vi "SmoothImage.vi"(0 "sector array in":cdb[][](array[numeric]) format="%.2f", 1 "Override min fill?":bool, 2 "Av size":i32=3, 3 "Min value":dbl format="%.2f") -> (4 "Smoothed Median":dbl[][](array[numeric]) format="%.2f", 5 "Smoothed Sector w/Ave":cdb[][](array[numeric]) format="%.2f", 6 "Var Array":dbl[][](array[numeric]), 7 "Soothed Sector w/ Max neighbor":dbl[][](array[numeric]) format="%.2f")   [LabVIEW 2022 SP3]
uses:
  <vilib>/Analysis/NI_AALBase.lvlib
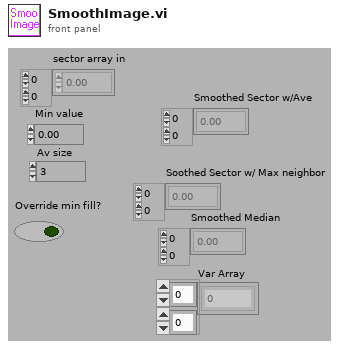
[diagram p1: front panel]
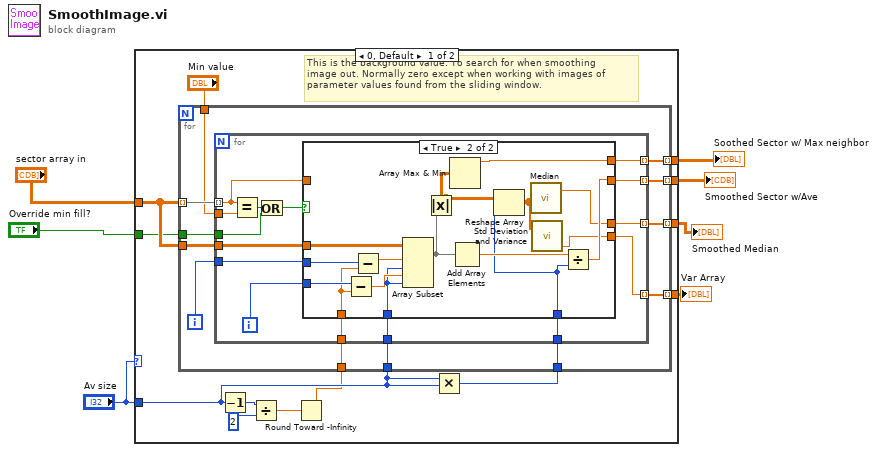
[diagram p0: block diagram]
diagram:
  n1 = case shown="0, Default" "Av size" {
    tunnel: "sector array in" -> [w20 w65]
    tunnel: [w19 w65] -> w6
    tunnel: [w18 w65] -> w5
    tunnel: "Av size" -> [w14 _]
    tunnel: "Override min fill?" -> [w11 _]
    tunnel: [w9 w65] -> w3
    tunnel: [w8 w65] -> w2
    frame 0, Default {
      # "This is the background value. To search for when smoothing\nimage out. Normally zero except when working with images of \nparameter values found from the sliding window."
      n2 = Decrement(x=w14) -> (x-1=w10:i32)
      n3 = Divide(x=w10, y=2) -> (x/y=w13:dbl)
      n4 = Round Toward -Infinity(1:w13) -> (0:w12:dbl)
      n5 = Multiply(x=w14, y=w14) -> (x*y=w16:i32)
      n6 = for {
        tunnel: w20 -> [w32] mode=indexing
        tunnel: [w31] -> w19 mode=indexing
        tunnel: w20 -> [w30]
        tunnel: [w28] -> w18 mode=indexing
        tunnel: "Min value" -> [w27]
        tunnel: w14 -> [w26]
        tunnel: w16 -> [w25]
        tunnel: w12 -> [w24]
        tunnel: w11 -> [w23]
        tunnel: [w22] -> w9 mode=indexing
        tunnel: [w21] -> w8 mode=indexing
        i -> [w29]
        n7 = for {
          tunnel: w32 -> [w47] mode=indexing
          tunnel: [w46] -> w31 mode=indexing
          tunnel: w30 -> [w45]
          tunnel: w29 -> [w44]
          tunnel: [w42] -> w28 mode=indexing
          tunnel: w27 -> [w41]
          tunnel: w26 -> [w40]
          tunnel: w25 -> [w39]
          tunnel: w24 -> [w38]
          tunnel: w23 -> [w35]
          tunnel: [w34] -> w22 mode=indexing
          tunnel: [w33] -> w21 mode=indexing
          i -> [w43]
          n8 = Equal?(x=w47, y=w41) -> (x = y?=w37:bool)
          n9 = Or(x=w37, y=w35) -> (x .or. y?=w36:bool)
          n10 = case shown="True" w36 {
            tunnel: [w48 w55] -> w46
            tunnel: w47 -> [w48 _]
            tunnel: w45 -> [_ w64]
            tunnel: w44 -> [_ w58]
            tunnel: w43 -> [_ w57]
            tunnel: [w48 w60] -> w42
            tunnel: w40 -> [_ w59]
            tunnel: w39 -> [_ w52]
            tunnel: w38 -> [_ w56]
            tunnel: [w48 w54] -> w34
            tunnel: [_ w50] -> w33
            frame False {
            }
            frame True {
              n11 = Subtract(x=w57, y=w56) -> (x-y=w62:dbl)
              n12 = Subtract(x=w58, y=w56) -> (x-y=w63:dbl)
              n13 = Array Subset(array=w64, index (row)=w63, length (row)=w59, index (col)=w62, length (col)=w59) -> (w53:cdb[][])
              n14 = Absolute Value(x=w53) -> (abs(x)=w49:dbl[][])
              n15 = Array Max & Min(array=w49) -> (max value=w60:dbl)  [unwired: 3 out]
              n16 = Add Array Elements(numeric array=w53) -> (sum=w61:cdb)
              n17 = Reshape Array(w49, w52) -> (w51:dbl[])
              n18 = call <vilib>:"Median.vi"("X"=w51) -> ("median"=w54:dbl)  [unwired: 1 out]
              n19 = call <vilib>:"Std Deviation and Variance.vi"("X"=w51) -> ("variance"=w50:dbl)  [unwired: 1 in, 2 out]
              n20 = Divide(x=w61, y=w52) -> (x/y=w55:cdb)
            }
          }
        }
      }
    }
    frame 1 {
    }
  }
  "Smoothed Sector w/Ave" <- w6
  "Soothed Sector w/ Max neighbor" <- w5
  "Smoothed Median" <- w3
  "Var Array" <- w2
